vi "OpenXL_WorkSheet.vi"   [LabVIEW 2015]
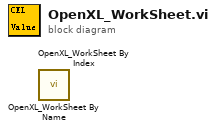
[diagram p0: block diagram]
diagram:
  n1 = call "OpenXL_WorkSheet By Name.vi"() -> ()  [unwired: 10 in, 2 out]
  n2 = call "OpenXL_WorkSheet By Index.vi"() -> ()  [unwired: 10 in, 2 out]
